vi "loadMTtempFile.vi"() -> ()   [LabVIEW 2012]
uses:
  <vilib>/addons/database/Connection.llb/DB Tools Open Connec (Path).vi
  <vilib>/addons/database/Connection.llb/Conn Execute.vi
  <vilib>/addons/database/Recordset.llb/Rec Fetch Recordset Data (R).vi
  <vilib>/addons/database/Recordset.llb/Rec Destroy - Connection.vi
  <vilib>/addons/database/_DB Variant To Data/Database Variant To Data.xnode
  <vilib>/addons/database/NI_Database_API.lvlib
panel:
  out "Output 2":string
  out "data":string
  in  "working directory":path=path "C:/temp/RunTemp"
  out "error out":errorcluster
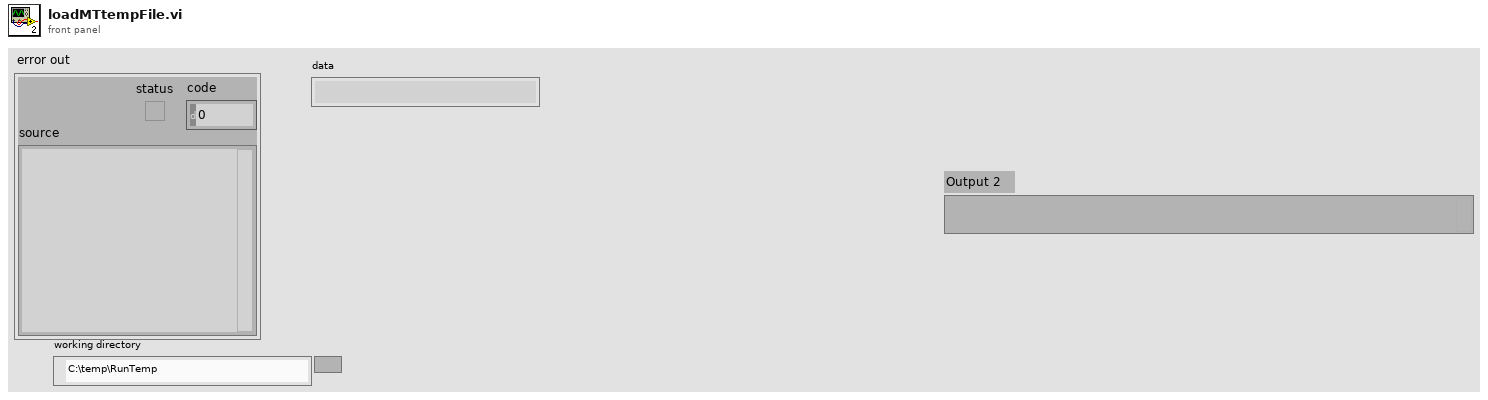
[diagram p1: front panel]
types:
  T1 = typedef "NI_Database_API.lvlib/Conn ObjectReference.ctl" = refnum<k1>
  T2 = typedef "NI_Database_API.lvlib/Rec ObjectReference.ctl" = refnum<k1>
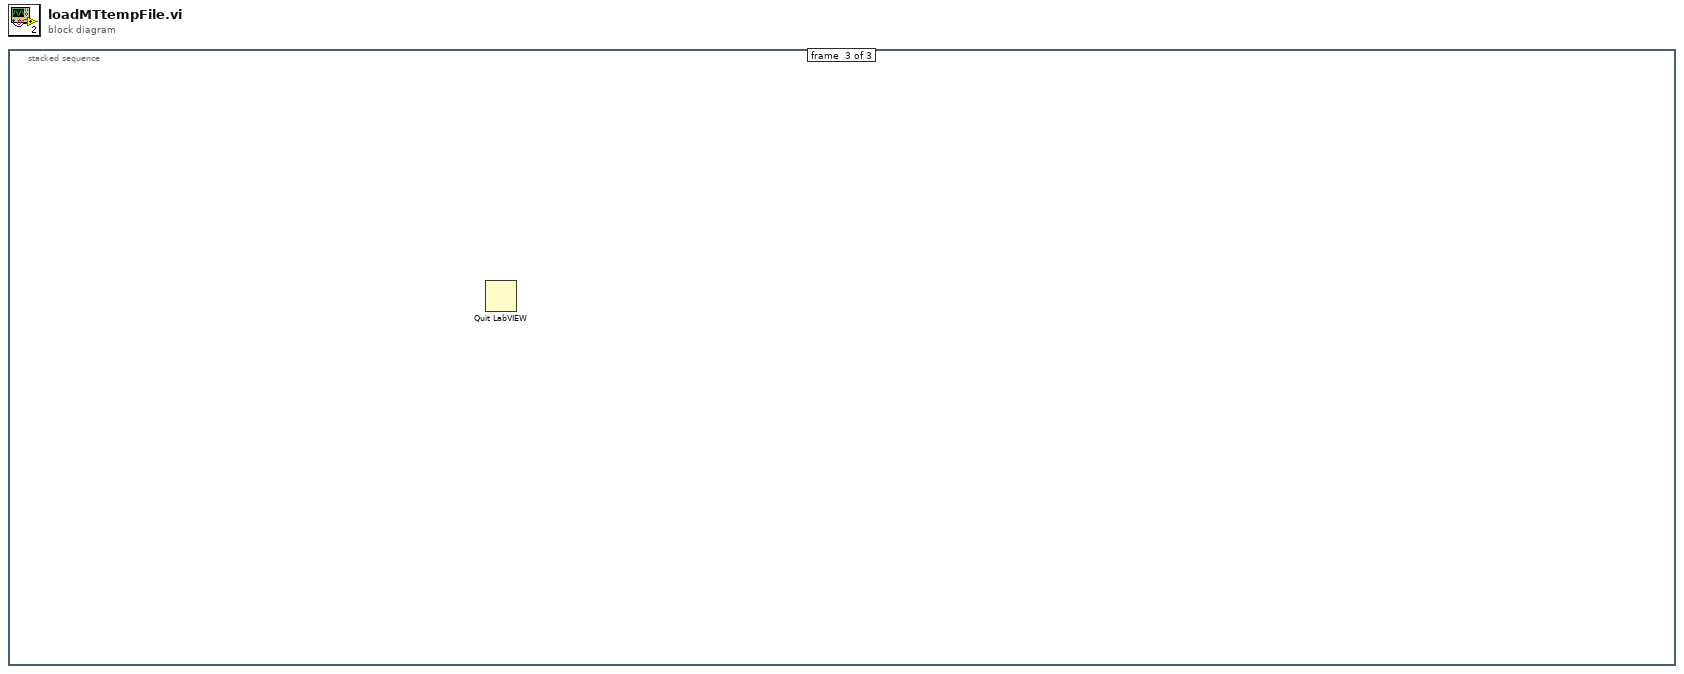
[diagram p0: block diagram]
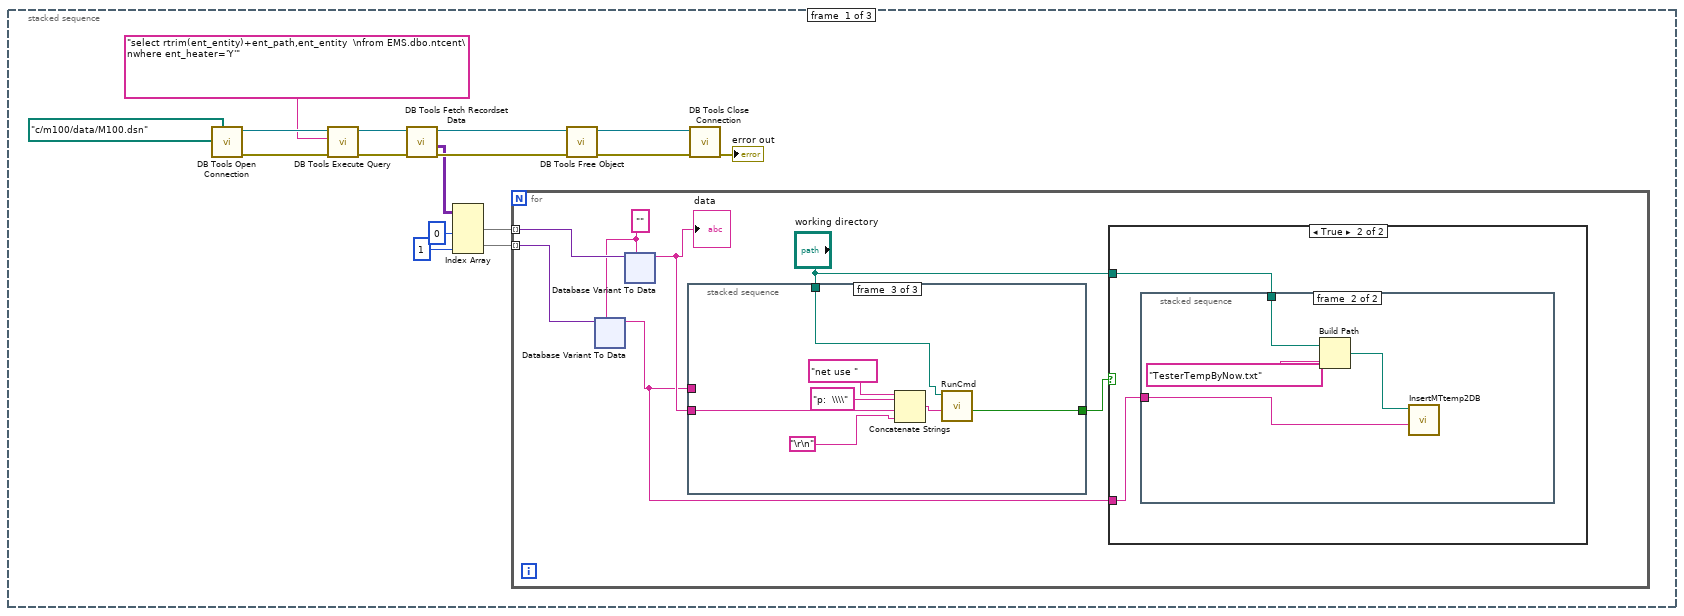
[diagram p2: hidden frame]
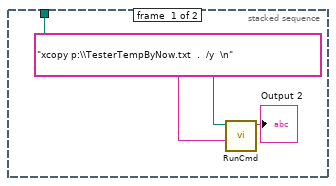
[diagram p4: hidden frame]
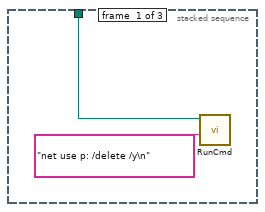
[diagram p5: hidden frame]
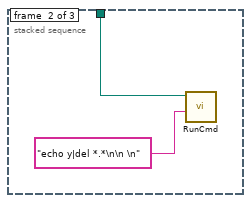
[diagram p6: hidden frame]
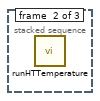
[diagram p7: hidden frame]
diagram:
  n1 = stacked-sequence {
    frame #0 {
      n2 = call-poly <vilib>:"DB Tools Open Connection.vi"("connection information"=path "c:/m100/data/M100.dsn") -> ("error out"=w12:errorcluster, "connection reference"=w16:T1)  [unwired: 7 in]
      n3 = call-poly <vilib>:"DB Tools Execute Query.vi"("error in (no error)"=w12, "SQL query"="select rtrim(ent_entity)+ent_path,ent_entity  \nfrom EMS.dbo.ntcent\nwhere ent_heater='Y'", "connection reference"=w16) -> ("error out"=w11:errorcluster, "recordset reference"=w15:T2)  [unwired: 5 in]
      n4 = call-poly <vilib>:"DB Tools Fetch Recordset Data.vi"("error in (no error)"=w11, "recordset reference"=w15) -> ("error out"=w10:errorcluster, "recordset data"=w5:variant[][], "recordset reference out"=w14:T2)  [unwired: 3 in]
      n5 = Index Array(array=w5, index (col) #1=0 ("disabled index (col)"), index (col) #2=1 ("index (col)")) -> (element #1=w3:variant[], element #2=w1:variant[])  [unwired: 2 in]
      n6 = for {
        tunnel: w3 -> [w23] mode=indexing
        tunnel: w1 -> [w21] mode=indexing
        w20 = ""
        n7 = xnode "Database Variant To Data"("database variant"=w21, "type"=w20) -> ("data"=w18:string)  [unwired: 1 in, 1 out]
        n8 = xnode "Database Variant To Data"("database variant"=w23, "type"=w20) -> ("data"=w22:string)  [unwired: 1 in, 1 out]
        "data" <- w22
        n9 = stacked-sequence {
          tunnel: "working directory" -> [w65 w67 w71]
          tunnel: w22 -> [_ _ w70]
          tunnel: w18 -> [_ _ _]
          tunnel: [_ _ w69] -> w17
          frame #0 {
            n10 = call "RunCmd.vi"("Cmd String"="net use p: /delete /y\n" ("string"), "working directory"=w65) -> ()  [unwired: 8 in, 2 out]
          }
          frame #1 {
            n11 = call "RunCmd.vi"("Cmd String"="echo y|del *.*\n\n \n" ("standard input"), "working directory"=w67) -> ()  [unwired: 8 in, 2 out]
          }
          frame #2 {
            n12 = Concatenate Strings("net use " ("string"), "p:  \\\\" ("string"), w70, "\r\n") -> (w75:string)
            n13 = call "RunCmd.vi"("Cmd String"=w75, "working directory"=w71) -> ("OK"=w69:bool)  [unwired: 8 in, 1 out]
          }
        }
        n14 = case shown="True" w17 {
          tunnel: "working directory" -> [_ w25]
          tunnel: w18 -> [_ w24]
          frame False {
          }
          frame True {
            n15 = stacked-sequence {
              tunnel: w25 -> [w27 w32]
              tunnel: w24 -> [_ w29]
              frame #0 {
                n16 = call "RunCmd.vi"("Cmd String"="xcopy p:\\TesterTempByNow.txt  .  /y  \n" ("string"), "working directory"=w27) -> ("Output"=→"Output 2":string)  [unwired: 8 in, 1 out]
              }
              frame #1 {
                n17 = Build Path(base path=w32, name or relative path="TesterTempByNow.txt") -> (appended path=w30:path)
                n18 = call "InsertMTtemp2DB.vi"("Entity"=w29, "file (use dialog)"=w30) -> ()  [unwired: 9 in, 1 out]
              }
            }
          }
        }
      }
      n19 = call-poly <vilib>:"DB Tools Free Object.vi"("error in (no error)"=w10, "recordset reference"=w14) -> ("error out"=w9:errorcluster, "connection reference"=w13:T1)  [unwired: 8 in]
      n20 = call <vilib>:"DB Tools Close Connection.vi"("error in (no error)"=w9, "connection reference"=w13) -> ("error out"=→"error out":errorcluster)  [unwired: 5 in]
    }
    frame #1 {
      n21 = call "runHTTemperature.vi"() -> ()  [unwired: 12 in]
    }
    frame #2 {
      n22 = Quit LabVIEW() -> ()  [unwired: 1 in]
    }
  }
